vi "GetText.vi"(8 "error in":errorcluster, 11 "node in":refnum<class "VI modification.lvclass">) -> (0 "error out":errorcluster, 1 "additional text":string, 2 "text":string, 3 "node out":refnum<class "VI modification.lvclass">, 4 "glyph":string)   [LabVIEW 2013, in "VI modification.lvclass"]
doc: "Returns the text representation of the node used for the tree control."
uses:
  VI modification.lvclass
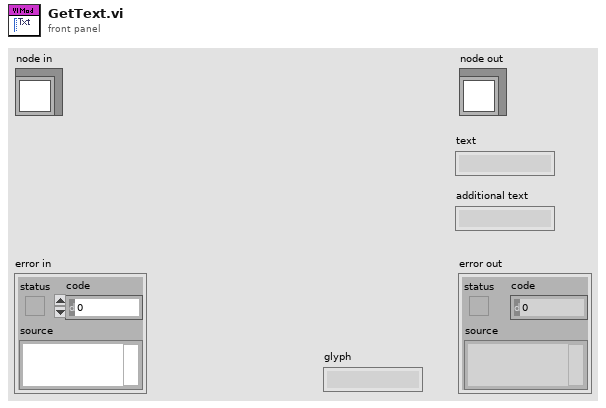
[diagram p1: front panel]
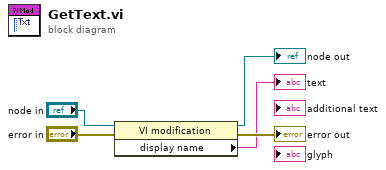
[diagram p0: block diagram]
diagram:
  n1 = property class="VI modification"(reference="node in", error in="error in") -> (reference out=→"node out":refnum<class "VI modification.lvclass">, error out=→"error out":errorcluster, "display name"=→"text":string)
